vi "Draw Valley.vi"(0 "Valley Points":T1[][](array[typedef])) -> (1 "Valley Basic":string="#.######\n#>>.<^<#\n#.<..<<#\n#>v.><>#\n#<^v^^>#\n######.#", 2 "Valley Colorful":u32[][](array[colorbox]))   [LabVIEW 2020, in "AoC 2022.lvlib"]
uses:
  AoC 2022.lvlib
  Valley Point.ctl
  Valley Item.ctl
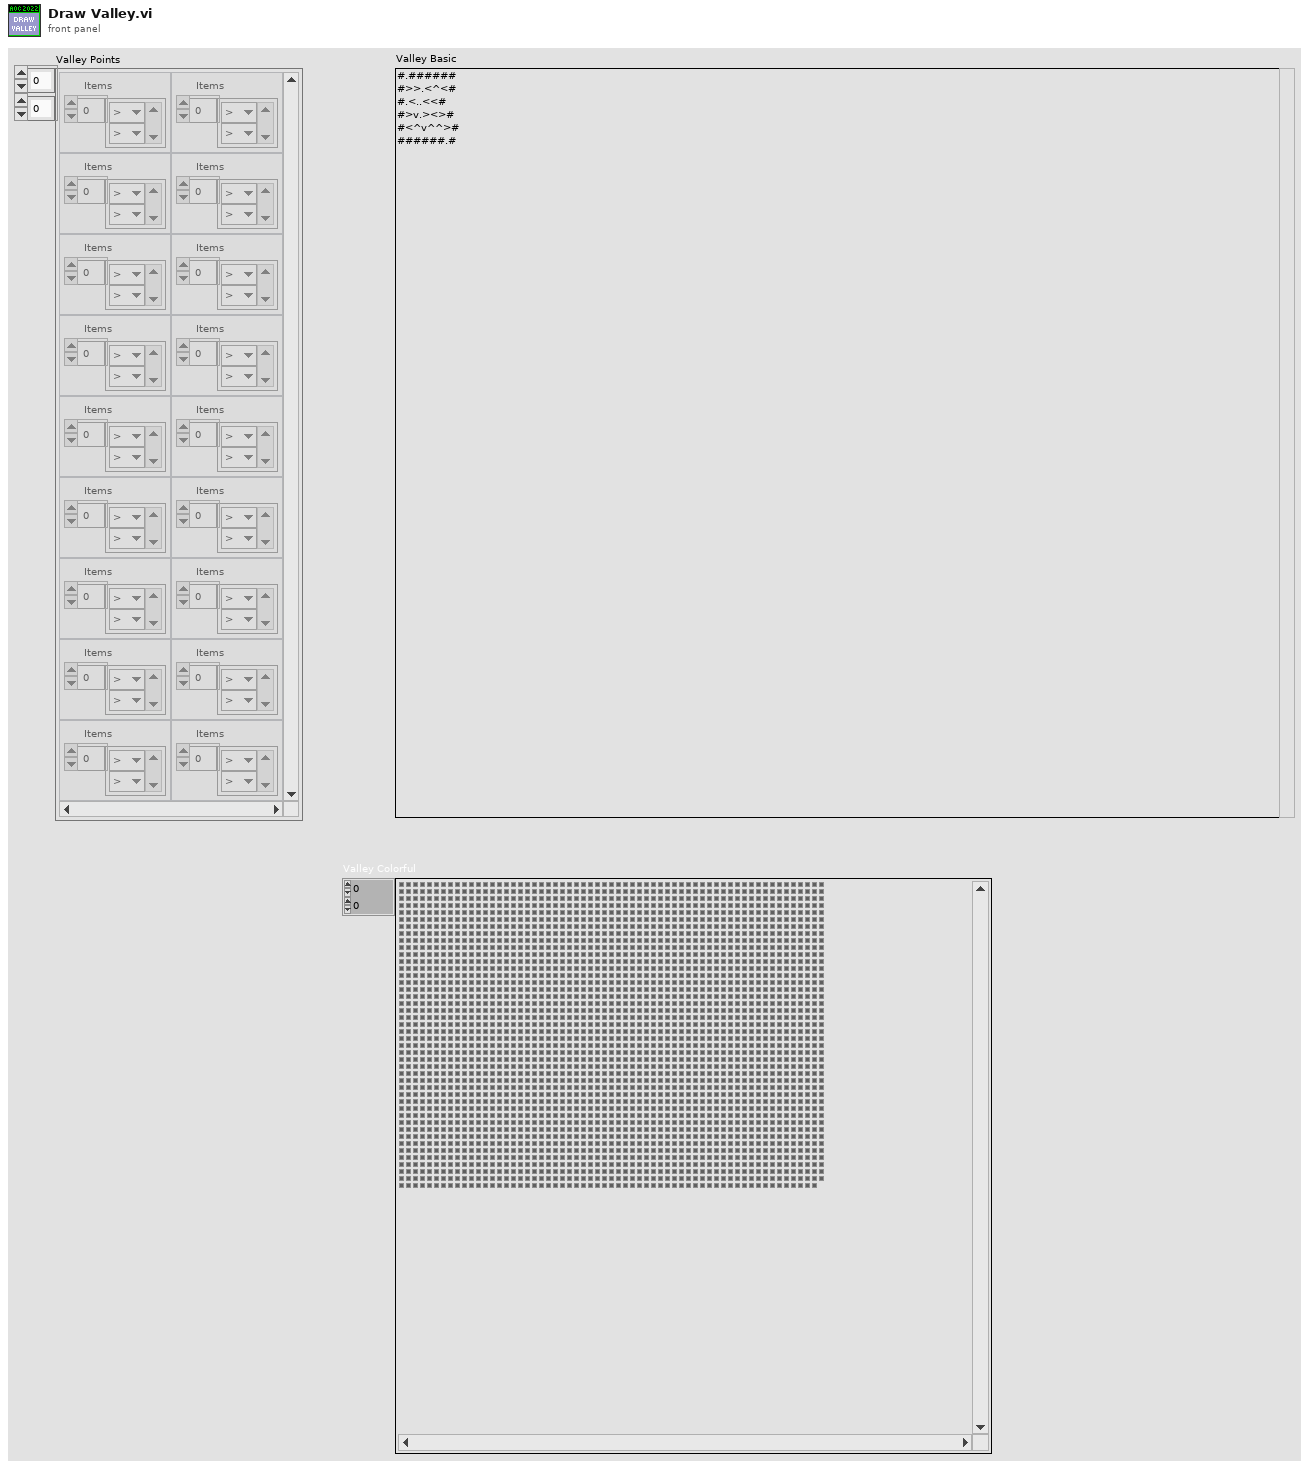
[diagram p1: front panel]
types:
  T1 = typedef "AoC 2022.lvlib/Valley Point.ctl" = cluster{"Items":T2[]}
  T2 = typedef "AoC 2022.lvlib/Valley Item.ctl" = enum16{"#", ".", ">", "<", "^", "v", "E"}
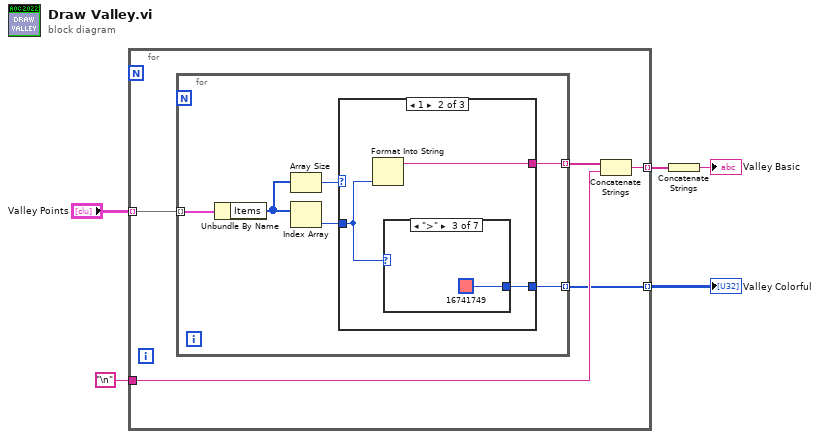
[diagram p0: block diagram]
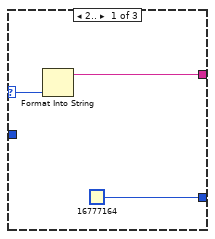
[diagram p2: hidden frame]
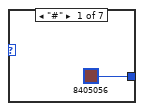
[diagram p3: hidden frame]
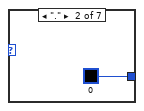
[diagram p4: hidden frame]
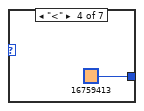
[diagram p5: hidden frame]
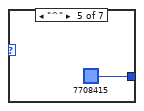
[diagram p6: hidden frame]
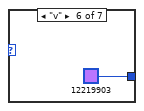
[diagram p7: hidden frame]
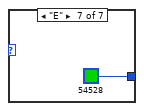
[diagram p8: hidden frame]
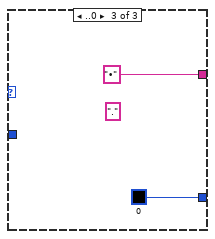
[diagram p9: hidden frame]
diagram:
  n1 = for {
    tunnel: "Valley Points" -> [w10] mode=indexing
    tunnel: "\n" -> [w8]
    tunnel: [w7] -> w4 mode=indexing
    tunnel: [w6] -> w1 mode=indexing
    n2 = for {
      tunnel: w10 -> [w16] mode=indexing
      tunnel: [w12] -> w9 mode=indexing
      tunnel: [w11] -> w6 mode=indexing
      n3 = Unbundle By Name(w16) -> ("Items"=w14:T2[])
      n4 = Array Size(array=w14) -> (size(s)=w15:i32)
      n5 = Index Array(array=w14) -> (element=w13:T2)  [unwired: 1 in]
      n6 = case shown="1" w15 {
        selector: w15 -> [w19 _ _]
        tunnel: w13 -> [_ w21 _]
        tunnel: [w18 w22 "•"] -> w12
        tunnel: [u32 16777164 w20 u32 0] -> w11
        frame 2.. {
          n7 = Format Into String(w19) -> (resulting string=w18:string)  [unwired: 3 in, 1 out]
        }
        frame 1 {
          n8 = Format Into String(w21) -> (resulting string=w22:string)  [unwired: 3 in, 1 out]
          n9 = case shown="\">\"" w21 {
            tunnel: [u32 8405056 u32 0 u32 16741749 u32 16759413 u32 7708415 u32 12219903 u32 54528] -> w20
            frame "#" {
            }
            frame "." {
            }
            frame ">" {
            }
            frame "<" {
            }
            frame "^" {
            }
            frame "v" {
            }
            frame "E" {
            }
          }
        }
        frame ..0 {
          (unwired) "."
        }
      }
    }
    n10 = Concatenate Strings(w9, w8) -> (w7:string)
  }
  "Valley Colorful" <- w1
  n11 = Concatenate Strings(w4) -> (→"Valley Basic":string)
